vi "Update Preview.vi"(8 "error in (no error)":errorcluster, 11 "ElementEditorPanel in":refnum<class "ElementEditorPanel.lvclass">) -> (0 "error out":errorcluster, 3 "ElementEditorPanel out":refnum<class "ElementEditorPanel.lvclass">)   [LabVIEW 2020, in "VolatusGUIEditorCore.lvlib" / "ElementEditorPanel.lvclass"]
uses:
  ElementEditorPanel.lvclass
  VolatusGUIEditorCore/Update Preview Data.ctl
  ElementEditorPanel.lvclass/ElementEditorPanel.ctl
  VolatusGUIEditorCore/VolatusGUIEditorCore.lvlib
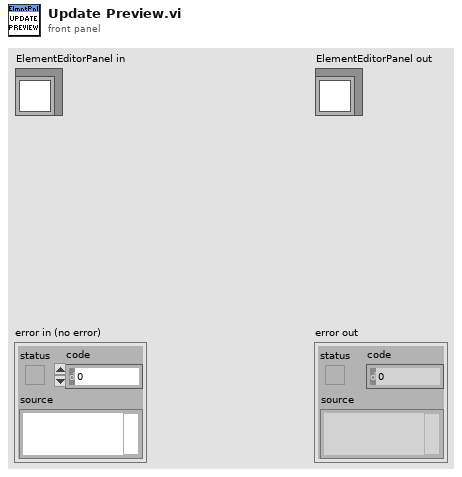
[diagram p1: front panel]
types:
  T1 = typedef "VolatusGUIEditorCore.lvlib/Update Preview Data.ctl" = cluster{"Unused":bool}
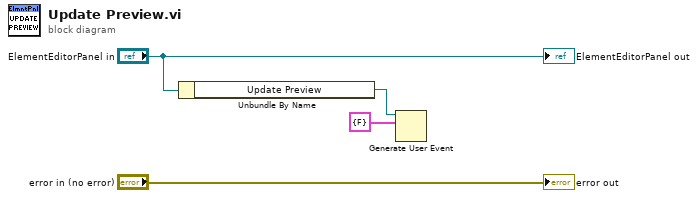
[diagram p0: block diagram]
diagram:
  n1 = Unbundle By Name("ElementEditorPanel in") -> ("Update Preview"=w2:refnum<user-event>)
  n2 = Generate User Event(user event=w2, event data cluster=T1 {"Unused"=FALSE} ("event data")) -> ()  [unwired: 2 in, 2 out]
  "error out" <- "error in (no error)"
  "ElementEditorPanel out" <- "ElementEditorPanel in"
